vi "Transceiver Thread.Transfer Group.Return.vi"(8 "error in (no error)":errorcluster, 10 "Transfer Group":refnum<class "Transfer Group.lvclass">, 11 "Transceiver Thread in":refnum<class "Transceiver Thread.lvclass">) -> (0 "error out":errorcluster, 3 "Transceiver Thread out":refnum<class "Transceiver Thread.lvclass">)   [LabVIEW 2017, in "DSF Core.lvlib" / "Transceiver Thread.lvclass"]
uses:
  Transceiver Thread.lvclass
  Transfer/Transfer Group.lvclass
  Transfer/Transfer Group.lvclass/Transfer Group.ctl
  Debug/Debug Flags.lvclass/Debug Flags.ctl
  Debug/FIFO Flags.lvclass/FIFO Flags.ctl
  Timing/Timing.lvclass/Timing.ctl
  Transfer/Transfer Group.Get Return FIFO.vi
  Transfer/Transfer Group.Get Timing.vi
  Timing/Timing.Get Iteration.vi
  Transfer/Transfer Group.Get Debug Flags.vi
  Debug/Debug Flags.Get FIFO Flags.vi
  Debug/FIFO Flags.Get Infinite Timeouts.vi
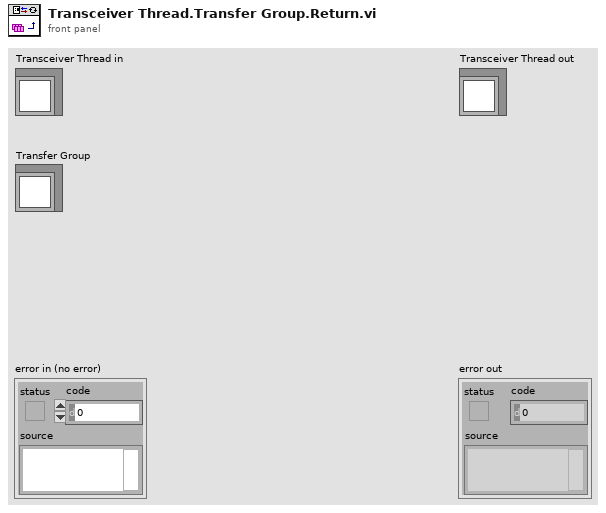
[diagram p1: front panel]
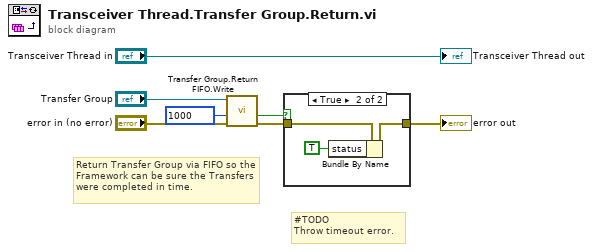
[diagram p0: block diagram]
diagram:
  # "#TODO\nThrow timeout error."
  # "Return Transfer Group via FIFO so the Framework can be sure the Transfers were completed in time."
  n1 = call "Transfer Group.Return FIFO.Write.vi"("error in (no error)"="error in (no error)", "timeout in ms (0)"=1000, "Transfer Group in"="Transfer Group") -> ("error out"=w3:errorcluster, "timed out?"=w4:bool)  [unwired: 6 in, 1 out]
  n2 = case shown="True" w4 {
    tunnel: w3 -> [w8 w11]
    tunnel: [w8 w9] -> w2
    frame False {
    }
    frame True {
      n3 = Bundle By Name(cluster=w11, "status"=TRUE) -> (w9:errorcluster)
    }
  }
  "error out" <- w2
  "Transceiver Thread out" <- "Transceiver Thread in"
